vi "Set DDS Boxing Style.vi"(10 "boxing":u32, 11 "channel_index":u8) -> ()   [LabVIEW 2021, in "vmmso.lvlib"]
doc: "DLL_API void WINAPI SetDDSBoxingStyle(unsigned char channel_index, unsigned int boxing);"
uses:
  vmmso.lvlib
  vmmso.dll
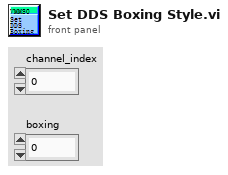
[diagram p1: front panel]
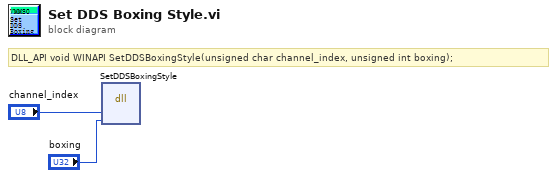
[diagram p0: block diagram]
diagram:
  # "DLL_API void WINAPI SetDDSBoxingStyle(unsigned char channel_index, unsigned int boxing);"
  n1 = dll-call lib="D:/labviewdemo/LabviewDemo 21/vmmso/vmmso.*" fn="SetDDSBoxingStyle"("channel_index"="channel_index", "boxing"="boxing") -> ()  [unwired: 6 in, 2 out]
